vi "MSScript_Act_Init.vi"(8 "error in (no error)":errorcluster, 9 "Listbox Ref":refnum<vi>, 10 "Script ctl ref":refnum<vi>) -> (0 "error out":errorcluster, 3 "MSScript out":refnum<class "MSScript.lvclass">)   [LabVIEW 2018, in "MSScript.lvclass"]
uses:
  MSScript.lvclass
  MSScript.lvclass/MSScript.ctl
  PublicSubVI/Class/DataXML/DataXML.lvclass
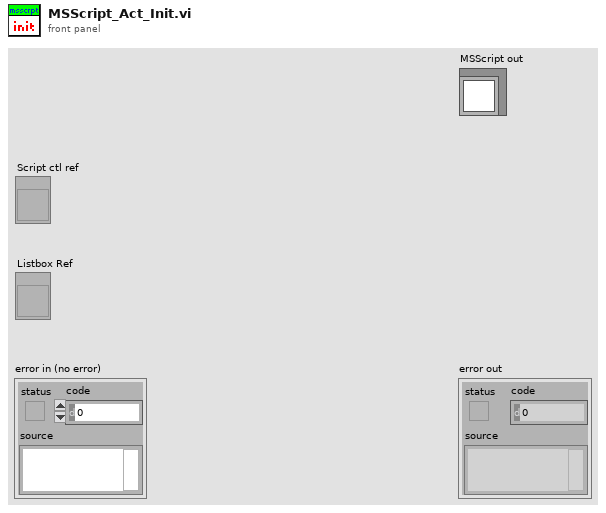
[diagram p1: front panel]
types:
  T1 = cluster{"VarName":string, "ArrayVariable":ext[]}[]
  T2 = cluster{"Type":string, "NAME":cluster{"STR":string, "Start":i32}, "PARAMs":cluster{"STR":string, "Start":i32}[]}[]
  T3 = cluster{"Colour":u32, "Italic":bool, "Bold":bool}
  T4 = enum8{"Enabled", "Disabled", "Disabled and Grayed Out"}
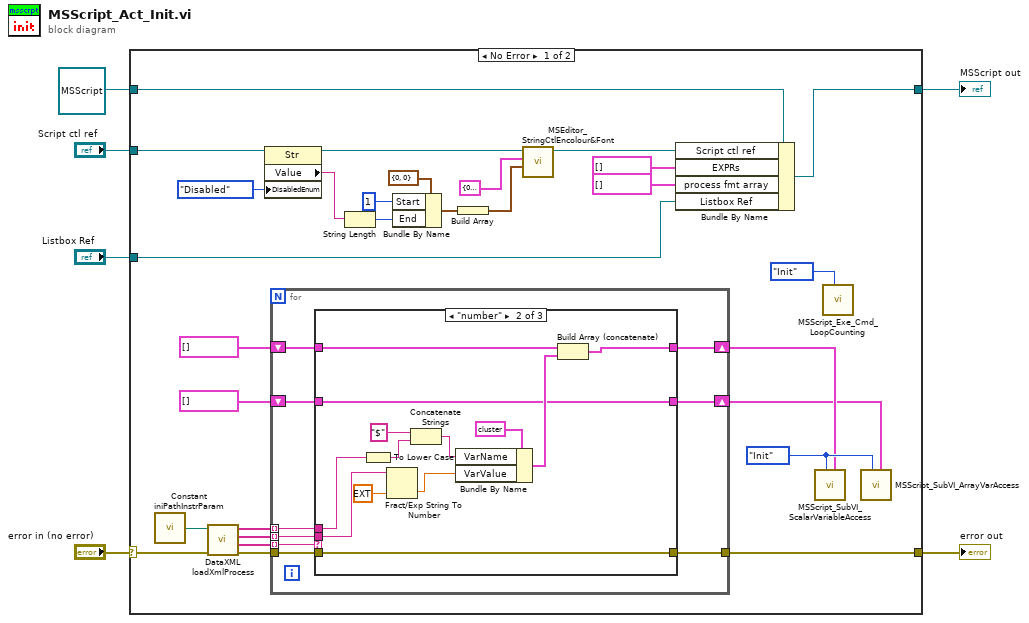
[diagram p0: block diagram]
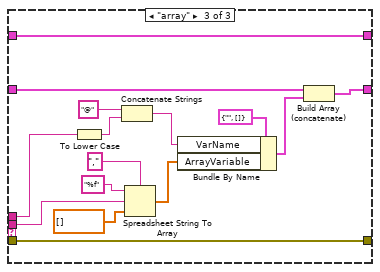
[diagram p3: hidden frame]
diagram:
  n1 = case shown="No Error" "error in (no error)" {
    selector: "error in (no error)" -> [w12 w77]
    tunnel: [w11 w77] -> w5
    tunnel: [w34 w76] -> w3
    tunnel: refnum<class "MSScript.lvclass"> refnum ("MSScript in") -> [w35 w76]
    tunnel: "Script ctl ref" -> [w27 _]
    tunnel: "Listbox Ref" -> [w25 _]
    frame No Error {
      w10 = enum16{"Init", "Write", "Read"}."Init" ("Function (Read)")
      n2 = call "Constant iniPathInstrParam.vi"() -> ("appended path"=w7:path)
      n3 = call "DataXML loadXmlProcess.vi"("error in (no error)"=w12, "xml_data_path"=w7) -> ("error IO"=w18:errorcluster, "type"=w15:string[], "value"=w16:string[], "name"=w17:string[])  [unwired: 6 in]
      n4 = property class="Str"(reference=w27, "DisabledEnum"=T4."Disabled" ("Disabled")) -> (reference out=w33:refnum<vi>, "Value"=w20:string)  [unwired: 1 in, 1 out]
      n5 = for {
        tunnel: w15 -> [w44] mode=indexing
        tunnel: w16 -> [w43] mode=indexing
        tunnel: w17 -> [w42] mode=indexing
        tunnel: w18 -> [w37]
        shift-right: [w39] -> w9
        shift-left: cluster{"VarName":string, "VarValue":ext}[] [] ("Init Data") -> [w41]
        shift-right: [w38] -> w8
        shift-left: T1 [] ("Init Data") -> [w40]
        tunnel: [w36] -> w11
        n6 = case shown="\"number\"" w44 {
          tunnel: w43 -> [_ w52 w75]
          tunnel: w42 -> [_ w50 w62]
          tunnel: w41 -> [w47 w57 w69]
          tunnel: w40 -> [w46 w54 w67]
          tunnel: [w47 w55 w69] -> w39
          tunnel: [w46 w54 w66] -> w38
          tunnel: w37 -> [w45 w53 w65]
          tunnel: [w45 w53 w65] -> w36
          frame Default {
          }
          frame "number" {
            n7 = To Lower Case(string=w50) -> (all lower case string=w49:string)
            n8 = Fract/Exp String To Number(string=w52, default (0 dbl)=ext 0.0 ("VarValue")) -> (number=w59:ext)  [unwired: 2 in, 1 out]
            n9 = Concatenate Strings("$" ("string"), w49) -> (w48:string)
            n10 = Bundle By Name(cluster=cluster{"VarName":string, "VarValue":ext} {"VarName"="", "VarValue"=0.0} ("VariableCluster"), "VarName"=w48, "VarValue"=w59) -> (w56:cluster{"VarName":string, "VarValue":ext})
            n11 = Build Array (concatenate)(w57, w56) -> (w55:cluster{"VarName":string, "VarValue":ext}[])
          }
          frame "array" {
            n12 = To Lower Case(string=w62) -> (all lower case string=w63:string)
            n13 = Concatenate Strings("@" ("string"), w63) -> (w61:string)
            n14 = Spreadsheet String To Array(delimiter (Tab)=",", format string="%f", spreadsheet string=w75, array type (2D Dbl)=ext[] [] ("ArrayVariable")) -> (array=w70:ext[])
            n15 = Bundle By Name(cluster=cluster{"VarName":string, "ArrayVariable":ext[]} {"VarName"="", "ArrayVariable"=[]} ("VariableCluster"), "VarName"=w61, "ArrayVariable"=w70) -> (w68:cluster{"VarName":string, "ArrayVariable":ext[]})
            n16 = Build Array (concatenate)(w67, w68) -> (w66:T1)
          }
        }
      }
      n17 = String Length(string=w20) -> (length=w19:i32)
      n18 = Bundle By Name(cluster=cluster{"Start":u32, "End":u32} {"Start"=0, "End"=0} ("SEL"), "Start"=u32 1 ("SEL.Start"), "End"=w19) -> (w30:cluster{"Start":u32, "End":u32})
      n19 = Build Array(w30) -> (w28:cluster{"Start":u32, "End":u32}[])
      n20 = call "MSEditor_StringCtlEncolour&Font.vi"("SELs"=w28, "TextProperties"=T3 {"Colour"=0, "Italic"=FALSE, "Bold"=FALSE}, "String ctl ref"=w33) -> ("String ctl ref out"=w32:refnum<vi>)  [unwired: 7 in, 1 out]
      n21 = Bundle By Name(cluster=w35, "Script ctl ref"=w32, "EXPRs"=T2 [], "process fmt array"=cluster{"Name":string, "Data":variant}[] [], "Listbox Ref"=w25) -> (w34:refnum<class "MSScript.lvclass">)
      n22 = call "MSScript_SubVI_ScalarVariableAccess.vi"("Init Data"=w9, "Function (Read)"=w10) -> ()  [unwired: 5 in, 3 out]
      n23 = call "MSScript_Exe_Cmd_LoopCounting.vi"("Function"=enum16{"Init", "LoopStart", "LoopEnd"}."Init") -> ()  [unwired: 9 in, 2 out]
      n24 = call "MSScript_SubVI_ArrayVarAccess.vi"("Init Data"=w8, "Function (Read)"=w10) -> ()  [unwired: 5 in, 3 out]
    }
    frame Error {
    }
  }
  "error out" <- w5
  "MSScript out" <- w3
